vi "DHT11_labview.vi"() -> ()   [LabVIEW 2025]
uses:
  <vilib>/Instr/_visa.llb/VISA Flush IO Buffer Mask.ctl
  <vilib>/Utility/error.llb/Trim Whitespace One-Sided.vi
  <vilib>/Instr/_visa.llb/VISA Configure Serial Port (Instr).vi
panel:
  out "Numeric":i32
  out "wilgotnoœæ liczba":dbl
  out "Wilgotnoœæ wykres":dbl(graph)
  out "Temperatura liczba":dbl
  out "Temperatura wykres":dbl(graph)
  out "wyœwietlanie danych":string
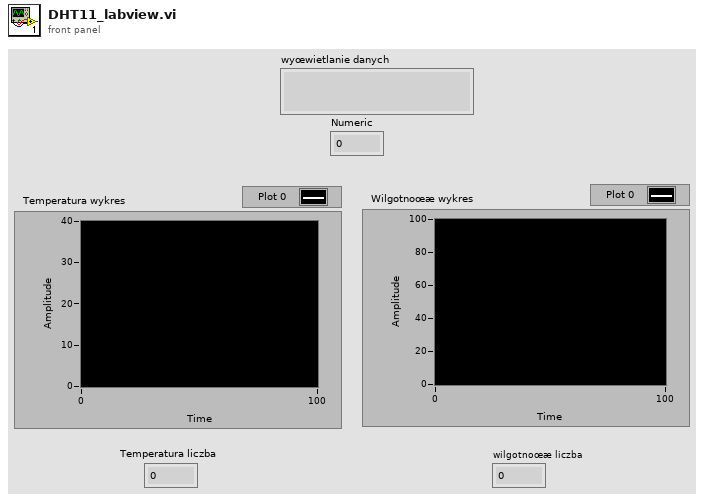
[diagram p1: front panel]
types:
  T1 = typedef "VISA Flush IO Buffer Mask.ctl" = u16
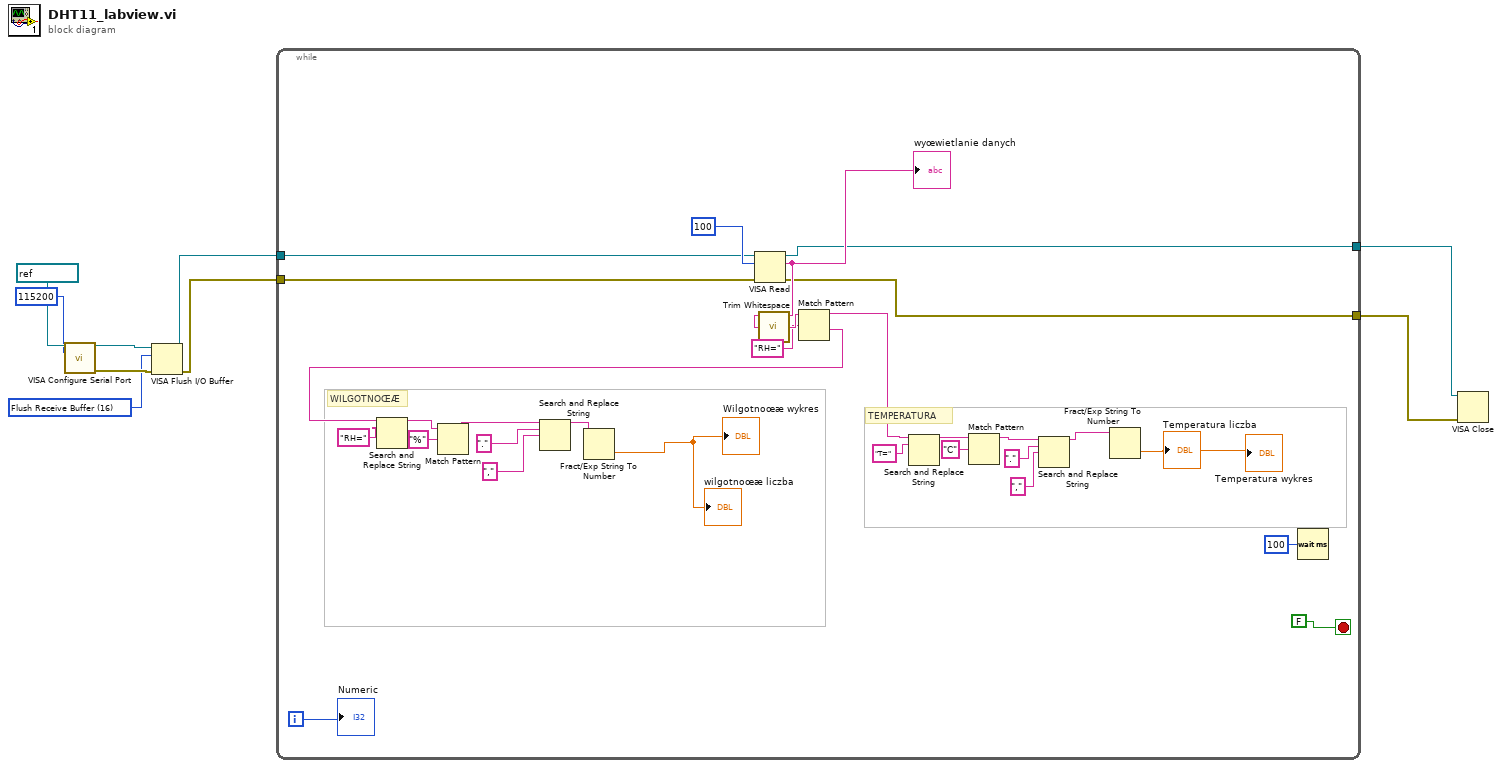
[diagram p0: block diagram]
diagram:
  w5 = T1 16 items=["Flush Receive Buffer"=16, "Write Transmit Buffer to Device"=32, "Flush Receive Buffer (No I/O)"=64, "Flush Transmit Buffer"=128] ("Mask")
  n1 = call-poly "VISA Configure Serial Port"("VISA resource name"=refnum<visa-resource-name> "COM7", "baud rate (9600)"=u32 115200) -> ("VISA resource name out"=w7:refnum<visa-resource-name>, "error out"=w6:errorcluster)  [unwired: 12 in]
  n2 = VISA Flush I/O Buffer(VISA resource name=w7, mask (16)=w5, error in (no error)=w6) -> (VISA resource name out=w3:refnum<visa-resource-name>, error out=w4:errorcluster)
  n3 = while {
    tunnel: w4 -> [w17]
    tunnel: w3 -> [w15]
    tunnel: [w14] -> w2
    tunnel: [w13] -> w1
    i -> [w11]
    stop <- FALSE stop-if-true
    # "WILGOTNOŒÆ"
    # "TEMPERATURA"
    n4 = VISA Read(VISA resource name=w15, byte count=u32 100, error in (no error)=w17) -> (VISA resource name out=w13:refnum<visa-resource-name>, read buffer=w27:string, error out=w14:errorcluster)  [unwired: 1 out]
    "wyœwietlanie danych" <- w27
    n5 = call <vilib>:"Trim Whitespace.vi"("string"=w27) -> ("trimmed string"=w28:string)  [unwired: 1 in]
    n6 = Match Pattern(string=w28, regular expression="RH=") -> (before substring=w29:string, after substring=w34:string)  [unwired: 1 in, 2 out]
    n7 = Search and Replace String(input string=w34, search string="RH=") -> (result string=w35:string)  [unwired: 6 in, 3 out]
    n8 = Match Pattern(string=w35, regular expression="%") -> (before substring=w36:string)  [unwired: 1 in, 3 out]
    n9 = Search and Replace String(input string=w36, search string=".", replace string="," ("replace string (\"\")")) -> (result string=w37:string)  [unwired: 5 in, 3 out]
    n10 = Fract/Exp String To Number(string=w37) -> (number=→"Wilgotnoœæ wykres" →"wilgotnoœæ liczba":dbl)  [unwired: 3 in, 1 out]
    n11 = Search and Replace String(input string=w29, search string="T=" ("replace string (\"\")")) -> (result string=w30:string)  [unwired: 6 in, 3 out]
    n12 = Match Pattern(string=w30, regular expression="C") -> (before substring=w31:string)  [unwired: 1 in, 3 out]
    n13 = Search and Replace String(input string=w31, search string=".", replace string="," ("replace string (\"\")")) -> (result string=w32:string)  [unwired: 5 in, 3 out]
    n14 = Fract/Exp String To Number(string=w32) -> (number=→"Temperatura wykres" →"Temperatura liczba":dbl)  [unwired: 3 in, 1 out]
    n15 = Wait (ms)(milliseconds to wait=u32 100) -> ()  [unwired: 1 out]
    "Numeric" <- w11
  }
  n16 = VISA Close(VISA resource name=w1, error in (no error)=w2) -> ()  [unwired: 1 out]
